vi "SetupDefault.vi"(8 "error in":errorcluster, 10 "Alias":string, 11 "SigGen_MXG in":refnum<class "SigGen_MXG.lvclass">) -> (0 "error out":errorcluster, 3 "SigGen_MXG out":refnum<class "SigGen_MXG.lvclass">)   [LabVIEW 2014, in "SigGen_MXG.lvclass"]
uses:
  SigGen_MXG.lvclass
  SigGen_MXG.lvclass/SigGen_MXG.ctl
  data/Agilent PSG MXG Series.lvlib
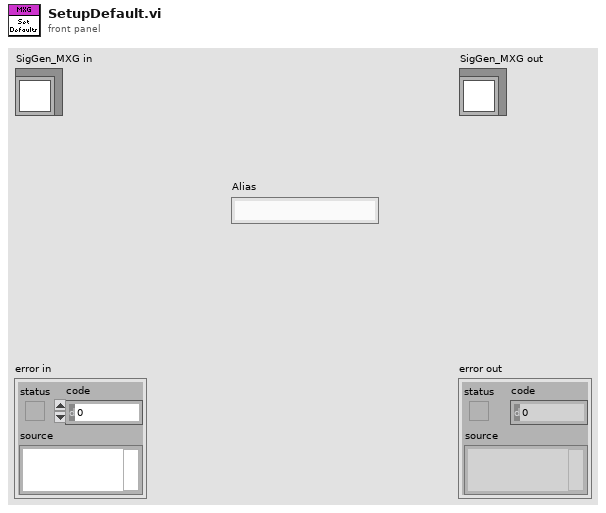
[diagram p1: front panel]
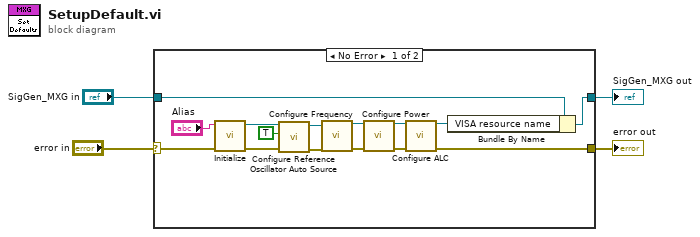
[diagram p0: block diagram]
diagram:
  n1 = case shown="No Error" "error in" {
    selector: "error in" -> [w10 w21]
    tunnel: "SigGen_MXG in" -> [w19 w20]
    tunnel: [w18 w20] -> w3
    tunnel: [w11 w21] -> w2
    frame No Error {
      n2 = call "Initialize.vi"("error in (no error)"=w10, "VISA resource name"="Alias") -> ("error out"=w8:errorcluster, "VISA resource name out"=w9:refnum<visa-resource-name>)  [unwired: 2 in, 6 out]
      n3 = call "Configure Reference Oscillator Auto Source.vi"("error in (no error)"=w8, "Auto Source (T:Enable)"=TRUE, "VISA resource name"=w9) -> ("error out"=w6:errorcluster, "VISA resource name out"=w7:refnum<visa-resource-name>)  [unwired: 7 in]
      n4 = call "Configure Frequency.vi"("VISA resource name"=w7, "error in (no error)"=w6) -> ("VISA resource name out"=w14:refnum<visa-resource-name>, "error out"=w15:errorcluster)  [unwired: 7 in, 5 out]
      n5 = call "Configure Power.vi"("VISA resource name"=w14, "error in (no error)"=w15) -> ("VISA resource name out"=w16:refnum<visa-resource-name>, "error out"=w17:errorcluster)  [unwired: 8 in, 4 out]
      n6 = call "Configure ALC.vi"("VISA resource name"=w16, "error in (no error)"=w17) -> ("VISA resource name out"=w12:refnum<visa-resource-name>, "error out"=w11:errorcluster)  [unwired: 6 in, 6 out]
      n7 = Bundle By Name(cluster=w19, "VISA resource name"=w12) -> (w18:refnum<class "SigGen_MXG.lvclass">)
    }
    frame Error {
    }
  }
  "error out" <- w2
  "SigGen_MXG out" <- w3
